vi "Untitled 4 (SubVI).vi"(10 "String in":string, 11 "String 2":string) -> (3 "String":string)   [LabVIEW 2017]
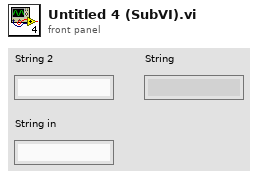
[diagram p1: front panel]
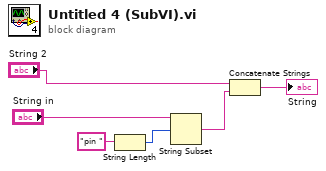
[diagram p0: block diagram]
diagram:
  n1 = String Length(string="pin ") -> (length=w6:i32)
  n2 = String Subset(string="String in", offset (0)=w6) -> (substring=w5:string)  [unwired: 1 in]
  n3 = Concatenate Strings("String 2", w5) -> (→"String":string)
